vi "Begin.vi"   [LabVIEW 2016]
doc: "Called before other user functions, this VI is expected to open initial I/O refnums, load in file data, and do all program initialization. Notice that the <B>error out</B> terminal is simply used for data flow. Wiring it to other structures or subVIs ensures that this VI runs first."
uses:
  <vilib>/Rock Robotics/WPI/Joystick/WPI_JoystickDeviceEnum.ctl
  <vilib>/Rock Robotics/SystemInterfaces/DIO/FPGA_DIOPWMChannel.ctl
  <vilib>/Rock Robotics/WPI/SafetyOutput/WPI_SafetyOutputConfigMenu.ctl
  <vilib>/Rock Robotics/WPI/Solenoid/WPI_SolenoidChannel.ctl
  <vilib>/Rock Robotics/WPI/MotorControl/WPI_MotorControlOpen VictorSP.vi
  External/2ndContollerStatus.vi
  <vilib>/Rock Robotics/WPI/RobotDrive/WPI_RobotDriveOpen2MotorWithVictorSP.vi
  <vilib>/Rock Robotics/WPI/Solenoid/WPI_SolenoidOpenSingle.vi
  <vilib>/Rock Robotics/WPI/RobotDrive/WPI_RobotDriveOpen4MotorWithVictorSP.vi
types:
  T1 = typedef "FPGA_DIOPWMChannel.ctl" = enum8{"PWM 0", "PWM 1", "PWM 2", "PWM 3", "PWM 4", "PWM 5", "PWM 6", "PWM 7", "PWM 8", "PWM 9", "PWM MXP 0", "PWM MXP 1", "PWM MXP 2", "PWM MXP 3", "PWM MXP 4", "PWM MXP 5", "PWM MXP 6", "PWM MXP 7", "PWM MXP 8", "PWM MXP 9", "Invalid"}
  T2 = typedef "WPI_SolenoidChannel.ctl" = enum8{"Solenoid 0", "Solenoid 1", "Solenoid 2", "Solenoid 3", "Solenoid 4", "Solenoid 5", "Solenoid 6", "Solenoid 7", "Invalid"}
  T3 = typedef "WPI_SafetyOutputConfigMenu.ctl" = enum16{"Enable", "Disable"}
  T4 = typedef "WPI_JoystickDeviceEnum.ctl" = enum16{"USB 0", "USB 1", "USB 2", "USB 3", "USB 4", "USB 5"}
  T5 = typedef "WPI_JoystickDevRef.ctl" = cluster{"Device":T4}
  T6 = typedef "WPI_SolenoidDevRef.ctl" = cluster{"DevStatus":errorcluster, "Pneumatics Control Module":u8, "Forward Solenoid Channel":T2, "Reverse Solenoid Channel":T2}
  T7 = typedef "WPI_MotorControlDeviceRef.ctl" = cluster{"DeviceStatus":errorcluster, "Type":T8, "PWM":cluster{"PWM Channel":T1, "DeadBand":T9}, "CAN":cluster{"Device Number":u8, "SetOutput VI Ref":variant, "GetOutput VI Ref":variant, "Enable VI Ref":variant, "Disable VI Ref":variant, "Data":variant}, "Invert":bool}
  T8 = typedef "WPI_MotorControlType.ctl" = enum16{"PWM", "CAN"}
  T9 = typedef "WPI_PWMDeadband.ctl" = cluster{"Name":string, "maxPositivePwm":i32, "minPositivePwm":i32, "centerPwm":i32, "maxNegativePwm":i32, "minNegativePwm":i32, "angularRange":u16}
  T10 = typedef "WPI_RobotDriveDevRef.ctl" = cluster{"DevStatus":errorcluster, "Motors[]":T7[], "Square Inputs":bool, "Max Output":dbl}
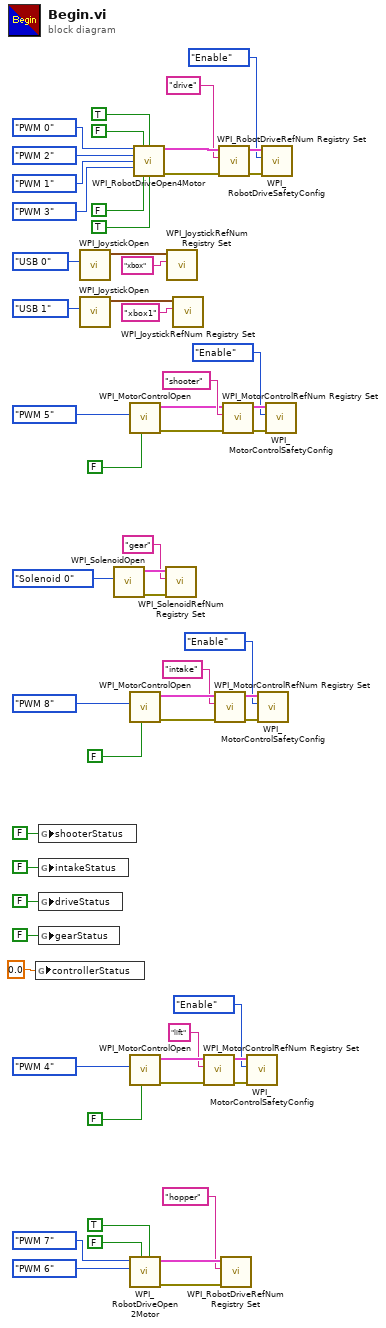
[diagram p0: block diagram]
diagram:
  n1 = global write "2ndContollerStatus.vi" "controllerStatus"(0.0 ("controllerStatus")) -> ()
  n2 = global write "2ndContollerStatus.vi" "shooterStatus"(FALSE ("shooterStatus")) -> ()
  n3 = global write "2ndContollerStatus.vi" "intakeStatus"(FALSE ("intakeStatus")) -> ()
  n4 = global write "2ndContollerStatus.vi" "driveStatus"(FALSE ("driveStatus")) -> ()
  n5 = global write "2ndContollerStatus.vi" "gearStatus"(FALSE ("gearStatus")) -> ()
  n6 = call <vilib>:"WPI_JoystickOpen.vi"("JoystickDevice"=WPI_JoystickDeviceEnum."USB 0") -> ("JoystickDevRef"=w53:T5)  [unwired: 10 in]
  n7 = call <vilib>:"WPI_JoystickOpen.vi"("JoystickDevice"=WPI_JoystickDeviceEnum."USB 1") -> ("JoystickDevRef"=w31:T5)  [unwired: 10 in]
  n8 = call-poly <vilib>:"WPI_SolenoidOpen.vi"("Solenoid Channel"=WPI_SolenoidChannel."Solenoid 0") -> ("error out"=w10:errorcluster, "SolenoidDevRef"=w11:T6)  [unwired: 9 in]
  n9 = call-poly <vilib>:"WPI_MotorControlOpen.vi"("Invert"=FALSE, "PWM Channel"=FPGA_DIOPWMChannel."PWM 5") -> ("error out"=w45:errorcluster, "MotorControlDeviceRef"=w46:T7)  [unwired: 8 in]
  n10 = call-poly <vilib>:"WPI_MotorControlOpen.vi"("Invert"=FALSE, "PWM Channel"=FPGA_DIOPWMChannel."PWM 8") -> ("error out"=w38:errorcluster, "MotorControlDeviceRef"=w39:T7)  [unwired: 8 in]
  n11 = call-poly <vilib>:"WPI_MotorControlOpen.vi"("Invert"=FALSE, "PWM Channel"=FPGA_DIOPWMChannel."PWM 4") -> ("error out"=w26:errorcluster, "MotorControlDeviceRef"=w27:T7)  [unwired: 8 in]
  n12 = call-poly <vilib>:"WPI_RobotDriveOpen2Motor.vi"("Right Motor Inverted"=TRUE, "Left Motor Inverted"=FALSE, "Right Motor"=FPGA_DIOPWMChannel."PWM 6" ("PWM Channel"), "Left Motor"=FPGA_DIOPWMChannel."PWM 7") -> ("error out"=w17:errorcluster, "RobotDriveDevRef"=w18:T10)  [unwired: 6 in]
  n13 = call-poly <vilib>:"WPI_RobotDriveOpen4Motor.vi"("Rear Left Motor"=FPGA_DIOPWMChannel."PWM 0", "Rear Left Motor Inverted"=FALSE, "Rear Right Motor Inverted"=TRUE, "Rear Right Motor"=FPGA_DIOPWMChannel."PWM 2", "Front Left Motor"=FPGA_DIOPWMChannel."PWM 1", "Front Right Motor"=FPGA_DIOPWMChannel."PWM 3", "Front Left Motor Inverted"=FALSE, "Front Right Motor Inverted"=TRUE) -> ("RobotDriveDevRef"=w60:T10, "error out"=w59:errorcluster)  [unwired: 6 in]
  n14 = call <vilib>:"WPI_SolenoidRefNum Registry Set.vi"("error in (no error)"=w10, "refnum name"="gear", "SolenoidDevRef"=w11) -> ()  [unwired: 7 in, 2 out]
  n15 = call <vilib>:"WPI_JoystickRefNum Registry Set.vi"("refnum name"="xbox", "JoystickDevRef"=w53) -> ()  [unwired: 8 in, 2 out]
  n16 = call <vilib>:"WPI_JoystickRefNum Registry Set.vi"("refnum name"="xbox1", "JoystickDevRef"=w31) -> ()  [unwired: 8 in, 2 out]
  n17 = call <vilib>:"WPI_MotorControlRefNum Registry Set.vi"("error in (no error)"=w26, "refnum name"="lift", "MotorControlDevRef"=w27) -> ("error out"=w23:errorcluster, "MotorControlDevRef"=w24:T7)  [unwired: 7 in]
  n18 = call <vilib>:"WPI_MotorControlRefNum Registry Set.vi"("error in (no error)"=w38, "refnum name"="intake", "MotorControlDevRef"=w39) -> ("error out"=w35:errorcluster, "MotorControlDevRef"=w36:T7)  [unwired: 7 in]
  n19 = call <vilib>:"WPI_RobotDriveRefNum Registry Set.vi"("error in (no error)"=w59, "refnum name"="drive", "RobotDriveDevRef"=w60) -> ("error out"=w56:errorcluster, "RobotDriveDevRef"=w57:T10)  [unwired: 7 in]
  n20 = call <vilib>:"WPI_RobotDriveRefNum Registry Set.vi"("error in (no error)"=w17, "refnum name"="hopper", "RobotDriveDevRef"=w18) -> ()  [unwired: 7 in, 2 out]
  n21 = call <vilib>:"WPI_MotorControlRefNum Registry Set.vi"("error in (no error)"=w45, "refnum name"="shooter", "MotorControlDevRef"=w46) -> ("error out"=w42:errorcluster, "MotorControlDevRef"=w43:T7)  [unwired: 7 in]
  n22 = call <vilib>:"WPI_MotorControlSafetyConfig.vi"("error in (no error)"=w23, "mode"=WPI_SafetyOutputConfigMenu."Enable", "MotorControlDevRef"=w24) -> ()  [unwired: 7 in, 2 out]
  n23 = call <vilib>:"WPI_MotorControlSafetyConfig.vi"("error in (no error)"=w35, "mode"=WPI_SafetyOutputConfigMenu."Enable", "MotorControlDevRef"=w36) -> ()  [unwired: 7 in, 2 out]
  n24 = call <vilib>:"WPI_RobotDriveSafetyConfig.vi"("error in (no error)"=w56, "mode"=WPI_SafetyOutputConfigMenu."Enable", "RobotDriveDevRef"=w57) -> ()  [unwired: 7 in, 2 out]
  n25 = call <vilib>:"WPI_MotorControlSafetyConfig.vi"("error in (no error)"=w42, "mode"=WPI_SafetyOutputConfigMenu."Enable", "MotorControlDevRef"=w43) -> ()  [unwired: 7 in, 2 out]
